vi "Conf.vi"() -> ()   [LabVIEW 2015]
uses:
  <vilib>/Utility/config.llb/Write Key (String).vi
  <vilib>/Utility/config.llb/NI_LVConfig.lvlib
panel:
  out "Error Out":errorcluster
  in  "Error In":errorcluster
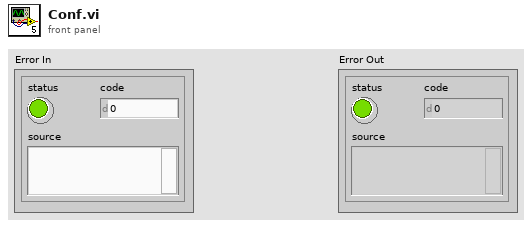
[diagram p1: front panel]
types:
  T1 = typedef "NI_LVConfig.lvlib/Config Data RefNum.ctl" = refnum<k1>
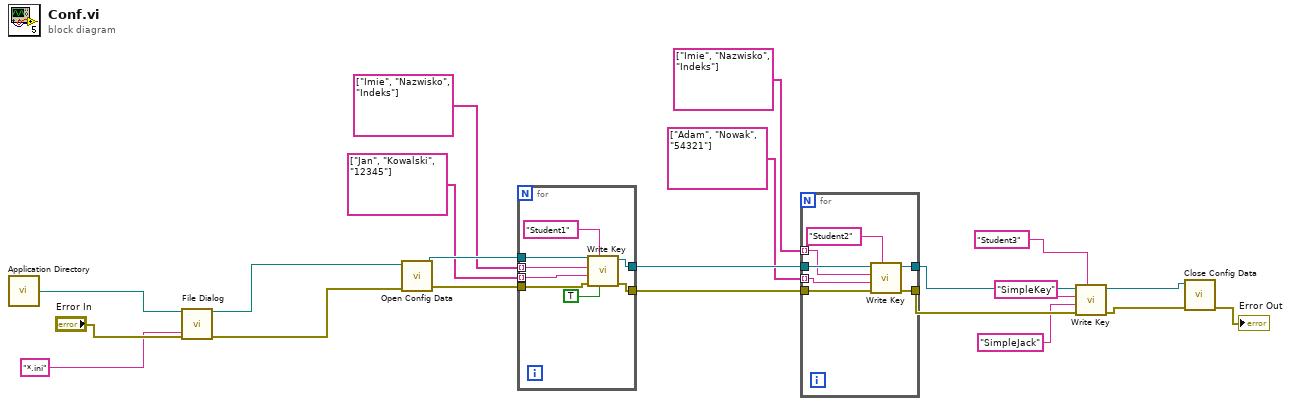
[diagram p0: block diagram]
diagram:
  n1 = call <vilib>:"Application Directory.vi"() -> ("Application Directory"=w12:path)
  n2 = call "File Dialog"("start path"=w12, "error in"="Error In", "pattern (all files)"="*.ini" ("prompt")) -> ("selected path"=w11:path, "error out"=w9:errorcluster)  [unwired: 9 in, 2 out]
  n3 = call <vilib>:"Open Config Data.vi"("error in (no error)"=w9, "configuration file path"=w11) -> ("error out"=w21:errorcluster, "refnum"=w20:T1)  [unwired: 7 in, 1 out]
  n4 = for {
    tunnel: w21 -> [w25]
    tunnel: w20 -> [w29]
    tunnel: string[] ["Imie", "Nazwisko", "Indeks"] -> [w27] mode=indexing
    tunnel: string[] ["Jan", "Kowalski", "12345"] -> [w26] mode=indexing
    tunnel: [w24] -> w17
    tunnel: [w23] -> w16
    n5 = call-poly <vilib>:"Write Key.vi"("write raw string? (F)"=TRUE, "section"="Student1", "error in (no error)"=w25, "value"=w26, "key"=w27, "refnum"=w29) -> ("error out"=w23:errorcluster, "refnum out"=w24:T1)  [unwired: 3 in, 1 out]
  }
  n6 = for {
    tunnel: w17 -> [w35]
    tunnel: w16 -> [w34]
    tunnel: string[] ["Adam", "Nowak", "54321"] -> [w33] mode=indexing
    tunnel: string[] ["Imie", "Nazwisko", "Indeks"] -> [w32] mode=indexing
    tunnel: [w31] -> w5
    tunnel: [w30] -> w6
    n7 = call-poly <vilib>:"Write Key.vi"("section"="Student2", "error in (no error)"=w34, "value"=w33, "key"=w32, "refnum"=w35) -> ("error out"=w31:errorcluster, "refnum out"=w30:T1)  [unwired: 4 in, 1 out]
  }
  n8 = call-poly <vilib>:"Write Key.vi"("section"="Student3", "error in (no error)"=w5, "value"="SimpleJack" ("key"), "key"="SimpleKey", "refnum"=w6) -> ("error out"=w2:errorcluster, "refnum out"=w1:T1)  [unwired: 4 in, 1 out]
  n9 = call <vilib>:"Close Config Data.vi"("error in (no error)"=w2, "refnum"=w1) -> ("error out"=→"Error Out":errorcluster)  [unwired: 8 in, 1 out]
